vi "Get Value (Integer).vi"(8 "error in (no error)":errorcluster, 10 "Feature":string, 11 "Camera in":refnum<class "Camera.lvclass">) -> (0 "error out":errorcluster, 2 "Value":i64, 3 "Camera":refnum<class "Camera.lvclass">)   [LabVIEW 2020, in "Camera.lvclass"]
uses:
  Camera.lvclass
  Camera.lvclass/Camera.ctl
  <vilib>/Utility/error.llb/Error Cluster From Error Code.vi
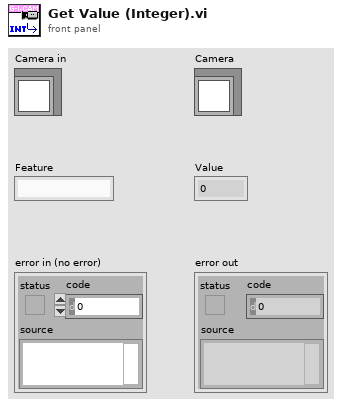
[diagram p1: front panel]
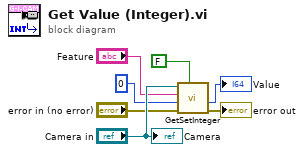
[diagram p0: block diagram]
diagram:
  n1 = call "GetSetInteger.vi"("Set?"=FALSE, "error in (no error)"="error in (no error)", "Value in"=i64 0, "Name"="Feature", "Camera in"="Camera in") -> ("error out"=→"error out":errorcluster, "Value out"=→"Value":i64)  [unwired: 5 in]
  "Camera" <- "Camera in"
